vi "Save Sensors.vi"(8 "error in (no error)":errorcluster, 10 "refnum":T1, 11 "Sensor List Class in":refnum<class "Sensor List Class.lvclass">) -> (0 "error out":errorcluster, 2 "refnum out":T1, 3 "Sensor List Class out":refnum<class "Sensor List Class.lvclass">)   [LabVIEW 2013, in "Sensor List Class.lvclass"]
uses:
  Sensor List Class.lvclass
  <vilib>/Utility/config.llb/Config Data RefNum.ctl
  Sensor DAO Class.lvclass
  Sensor List Class.lvclass/Sensor List Class.ctl
  Sensor DAO Class.lvclass/Sensor DAO Class.ctl
  <vilib>/Utility/config.llb/NI_LVConfig.lvlib
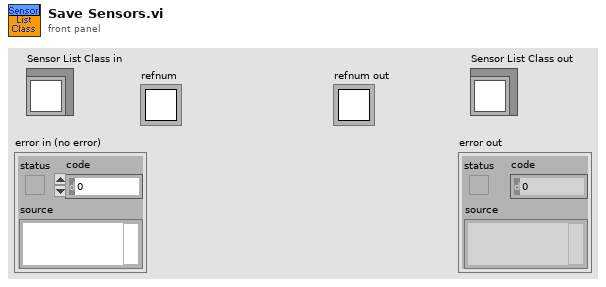
[diagram p1: front panel]
types:
  T1 = typedef "NI_LVConfig.lvlib/Config Data RefNum.ctl" = refnum<k1>
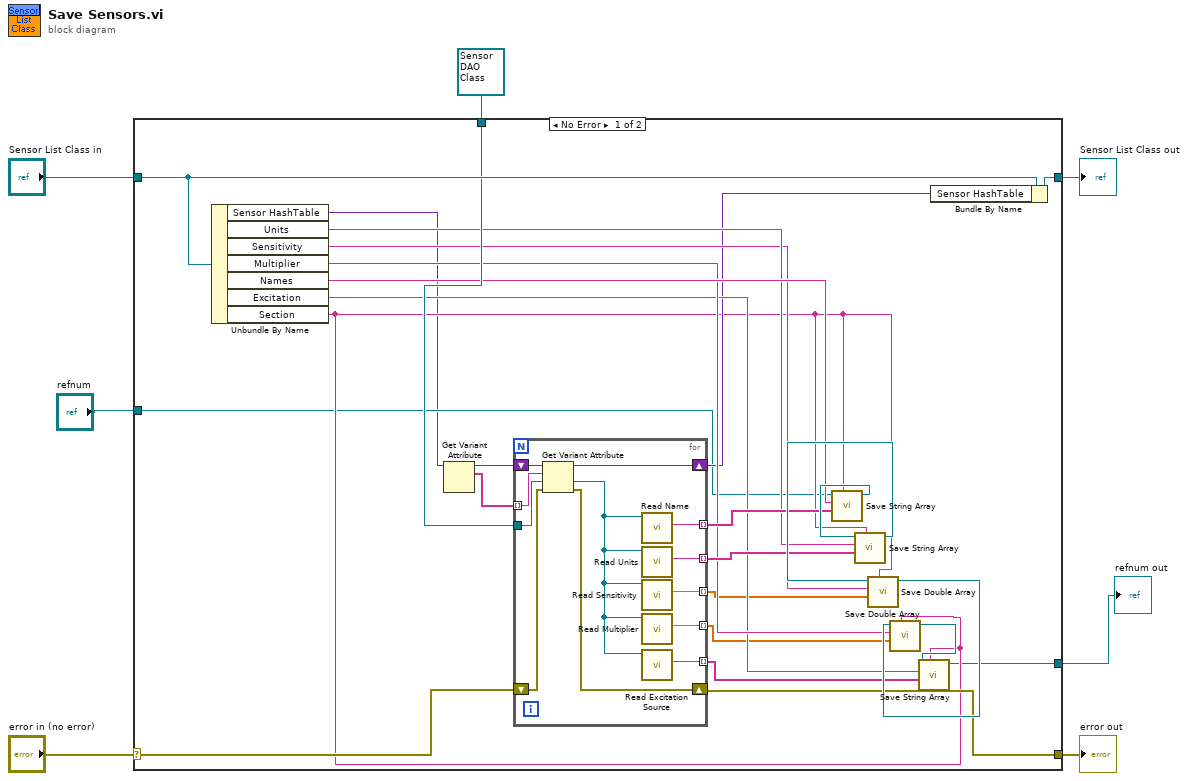
[diagram p0: block diagram]
diagram:
  n1 = case shown="No Error" "error in (no error)" {
    selector: "error in (no error)" -> [w21 w48]
    tunnel: [w20 w48] -> w6
    tunnel: [w23 w47] -> w4
    tunnel: "Sensor List Class in" -> [w24 w47]
    tunnel: refnum<class "Sensor DAO Class.lvclass"> refnum ("Sensor DAO In") -> [w22 _]
    tunnel: [w12 w46] -> w2
    tunnel: "refnum" -> [w11 w46]
    frame No Error {
      n2 = Unbundle By Name(w24) -> ("Sensor HashTable"=w10:variant, "Units"=w18:string, "Sensitivity"=w17:string, "Multiplier"=w16:string, "Names"=w19:string, "Excitation"=w15:string, "Section"=w13:string)
      n3 = Get Variant Attribute(Variant=w10) -> (duplicate Variant=w26:variant, names=w25:string[])  [unwired: 3 in, 2 out]
      n4 = for {
        tunnel: w25 -> [w44] mode=indexing
        shift-right: [w43] -> w14
        shift-left: w26 -> [w45]
        tunnel: w22 -> [w42]
        tunnel: [w41] -> w27 mode=indexing
        tunnel: [w40] -> w28 mode=indexing
        tunnel: [w39] -> w9 mode=indexing
        tunnel: [w38] -> w8 mode=indexing
        tunnel: [w36] -> w30 mode=indexing
        shift-right: [w34] -> w20
        shift-left: w21 -> [w35]
        n5 = Get Variant Attribute(Variant=w45, name=w44, default value (empty Variant)=w42, error in=w35) -> (duplicate Variant=w43:variant, value=w37:refnum<class "Sensor DAO Class.lvclass">, error out=w34:errorcluster)  [unwired: 1 out]
        n6 = call "Read Name.vi"("Sensor DAO Class in"=w37) -> ("Name"=w41:string)  [unwired: 8 in, 2 out]
        n7 = call "Read Units.vi"("Sensor DAO Class in"=w37) -> ("Units"=w40:string)  [unwired: 8 in, 2 out]
        n8 = call "Read Sensitivity.vi"("Sensor DAO Class in"=w37) -> ("Sensitivity"=w39:dbl)  [unwired: 8 in, 2 out]
        n9 = call "Read Multiplier.vi"("Sensor DAO Class in"=w37) -> ("Multiplier"=w38:dbl)  [unwired: 8 in, 2 out]
        n10 = call "Read Excitation Source.vi"("Sensor DAO Class in"=w37) -> ("Excitation Source"=w36:string)  [unwired: 8 in, 2 out]
      }
      n11 = call "Save String Array.vi"("section"=w13, "String Array In"=w27, "key"=w19, "refnum"=w11) -> ("refnum out"=w29:T1)  [unwired: 6 in, 1 out]
      n12 = call "Save String Array.vi"("section"=w13, "String Array In"=w28, "key"=w18, "refnum"=w29) -> ("refnum out"=w31:T1)  [unwired: 6 in, 1 out]
      n13 = call "Save Double Array.vi"("section"=w13, "Double Array In"=w9, "key"=w17, "refnum"=w31) -> ("refnum out"=w32:T1)  [unwired: 6 in, 1 out]
      n14 = call "Save Double Array.vi"("section"=w13, "Double Array In"=w8, "key"=w16, "refnum"=w32) -> ("refnum out"=w33:T1)  [unwired: 6 in, 1 out]
      n15 = call "Save String Array.vi"("section"=w13, "String Array In"=w30, "key"=w15, "refnum"=w33) -> ("refnum out"=w12:T1)  [unwired: 6 in, 1 out]
      n16 = Bundle By Name(cluster=w24, "Sensor HashTable"=w14) -> (w23:refnum<class "Sensor List Class.lvclass">)
    }
    frame Error {
    }
  }
  "error out" <- w6
  "Sensor List Class out" <- w4
  "refnum out" <- w2
